vi "YActor_Create.vi"(8 "ErrorIn":errorcluster, 11 "YActor in":refnum<class "YActor.lvclass">) -> (0 "ErrorOut":errorcluster, 3 "YActor out":refnum<class "YActor.lvclass">)   [LabVIEW 2021, in "YActor.lvclass"]
uses:
  YActor.lvclass
  private/CmdCtrl.ctl
  AsyncErrorHandling.ctl
  private/CallMode.ctl
  YActor.lvclass/YActor.ctl
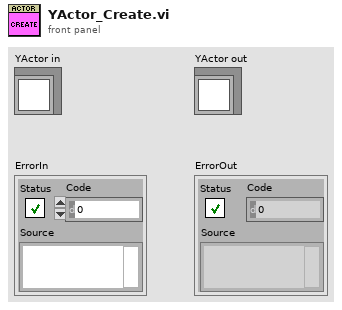
[diagram p1: front panel]
types:
  T1 = typedef "YActor.lvclass/AsyncErrorHandling.ctl" = enum16{"Return after executing sync command", "Return before executing sync command", "Don't return error"}
  T2 = typedef "YActor.lvclass/CmdCtrl.ctl" = cluster{"CmdData":variant, "CommandVI":string, "ReplyQ":i64, "Error":errorcluster, "Msg#":u32, "Async Error Handling":T1, "CallMode":T3, "Source":string}
  T3 = typedef "YActor.lvclass/CallMode.ctl" = enum16{"Standard", "Call&Collect"}
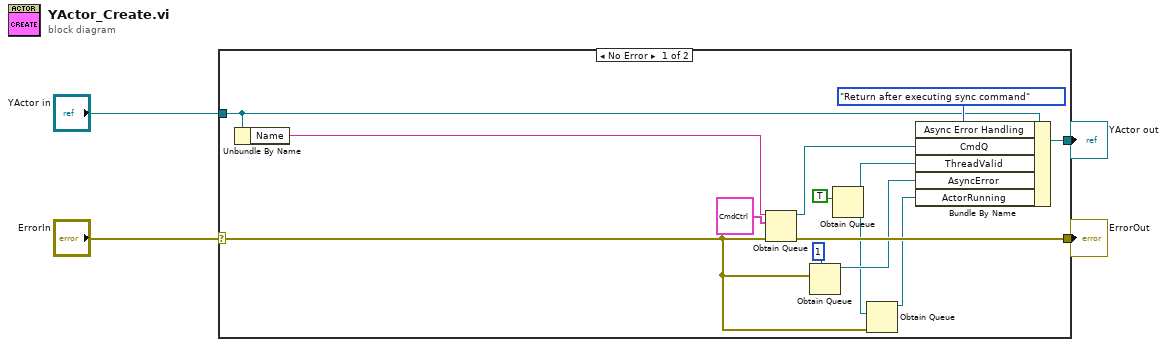
[diagram p0: block diagram]
diagram:
  n1 = case shown="No Error" "ErrorIn" {
    selector: "ErrorIn" -> [w16 w19]
    tunnel: [w17 w19] -> w3
    tunnel: "YActor in" -> [w6 w18]
    tunnel: [w12 w18] -> w2
    frame No Error {
      n2 = Unbundle By Name(w6) -> ("Name"=w5:string)
      n3 = Obtain Queue(name (unnamed)=w5, element data type=T2 {"CmdData"=variant(refnum<class> refnum), "CommandVI"="", "ReplyQ"=0, "Error"={"status"=FALSE, "code"=0, "source"=""}, "Msg#"=0, "Async Error Handling"=enum."Return after executing sync command", "CallMode"=enum."Standard", "Source"=""} ("CmdCtrl"), error in (no error)=w16) -> (queue out=w15:refnum<queue>, error out=w17:errorcluster)  [unwired: 2 in, 1 out]
      n4 = Obtain Queue(max queue size (-1, unlimited)=1, element data type=w16) -> (queue out=w9:refnum<queue>)  [unwired: 3 in, 2 out]
      n5 = Obtain Queue(element data type=TRUE) -> (queue out=w8:refnum<queue>)  [unwired: 4 in, 2 out]
      n6 = Obtain Queue(element data type=w8, error in (no error)=w16) -> (queue out=w7:refnum<queue>)  [unwired: 3 in, 2 out]
      n7 = Bundle By Name(cluster=w6, "Async Error Handling"=AsyncErrorHandling."Return after executing sync command", "CmdQ"=w15, "ThreadValid"=w8, "AsyncError"=w9, "ActorRunning"=w7) -> (w12:refnum<class "YActor.lvclass">)
    }
    frame Error {
    }
  }
  "ErrorOut" <- w3
  "YActor out" <- w2
